vi "Sorting_Single_Frame_Displ_2.vi"(0 "[IN] (X,Y,dX,dY)":dbl[][](array[numeric]), 2 "error IN":errorcluster) -> (3 "[OUT] Displ >1 Frame":dbl[][](array[numeric]), 4 "[OUT] Displ =1 Frame":dbl[][](array[numeric]), 6 "error OUT":errorcluster)   [LabVIEW 2017]
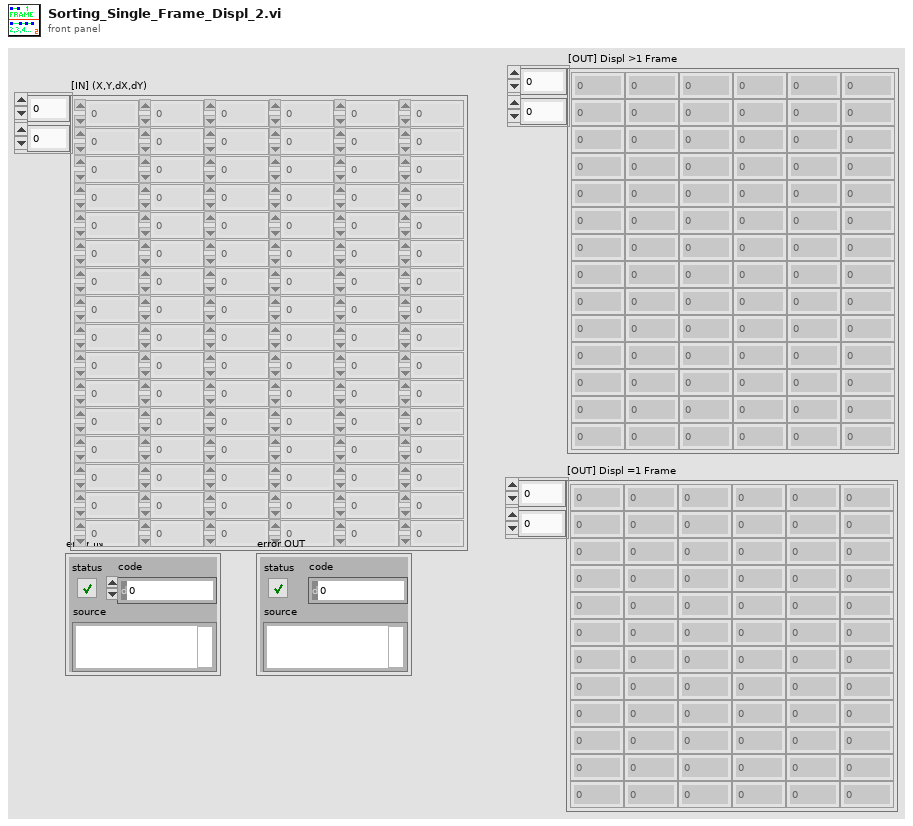
[diagram p1: front panel]
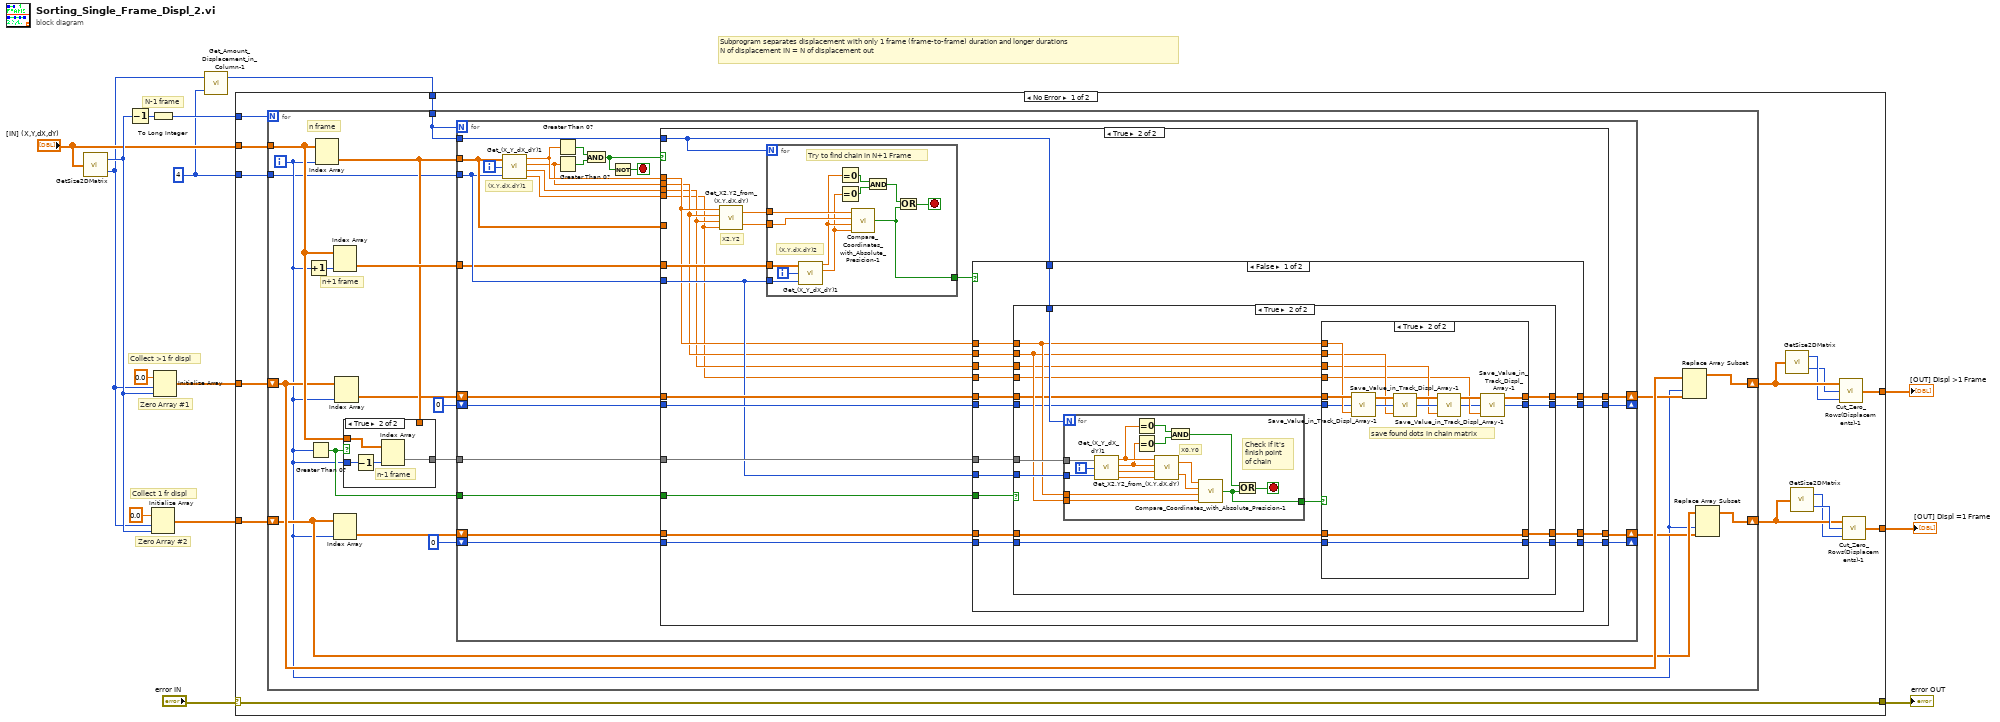
[diagram p0: block diagram]
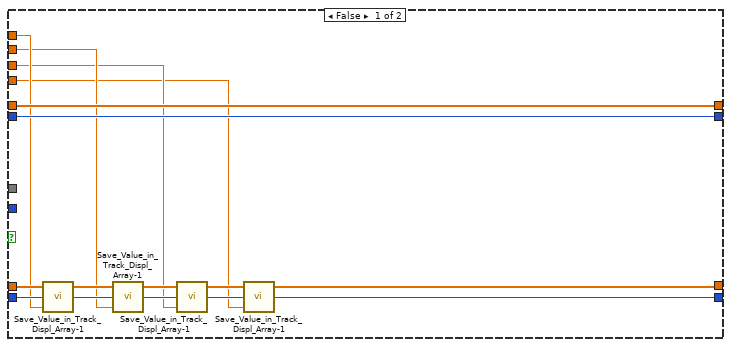
[diagram p4: hidden frame]
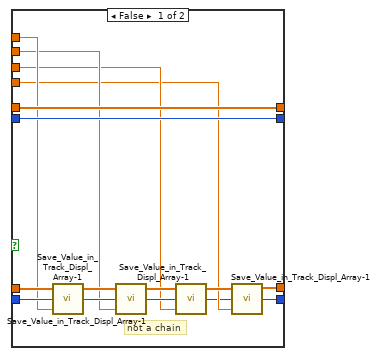
[diagram p5: hidden frame]
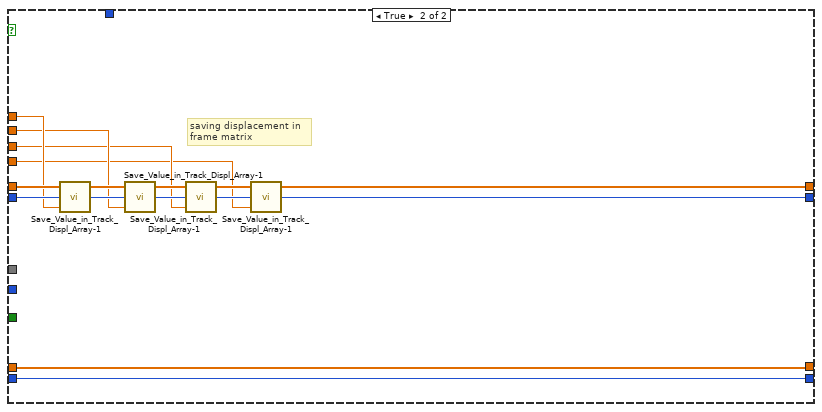
[diagram p6: hidden frame]
diagram:
  w4 = 4 ("y")
  # "Collect >1 fr displ"
  # "Collect 1 fr displ"
  # "Subprogram separates displacement with only 1 frame (frame-to-frame) duration and longer durations\nN of displacement IN = N of displacement out"
  # "Zero Array #2"
  # "Zero Array #1"
  # "N-1 frame"
  n1 = call "GetSize2DMatrix.vi"("Array IN (2D)"="[IN] (X,Y,dX,dY)") -> ("# Cols"=w10:i32, "# Rows"=w5:i32)
  n2 = Decrement(x=w10) -> (x-1=w15:i32)
  n3 = To Long Integer(number=w15) -> (32bit integer=w13:i32)
  n4 = Initialize Array(0.0 ("element"), w5, w10) -> (w9:dbl[][])
  n5 = Initialize Array(0.0 ("element"), w5, w10) -> (w12:dbl[][])
  n6 = call "Get_Amount_Displacement_in_Column-1.vi"("multiplier"=w4, "# Rows"=w5) -> ("Displ amount"=w3:i32)  [unwired: 1 out]
  n7 = case shown="No Error" "error IN" {
    selector: "error IN" -> [w16 w228]
    tunnel: w13 -> [w30 _]
    tunnel: w12 -> [w29 w226]
    tunnel: w9 -> [w28 w227]
    tunnel: "[IN] (X,Y,dX,dY)" -> [w21 _]
    tunnel: [w20 w226] -> w7
    tunnel: [w19 w227] -> w6
    tunnel: w4 -> [w18 _]
    tunnel: w3 -> [w17 _]
    tunnel: [w16 w228] -> w1
    frame No Error {
      n8 = for {
        N: w30 -> [_]
        shift-right: [w38] -> w27
        shift-left: w29 -> [w40]
        shift-right: [w34] -> w23
        shift-left: w28 -> [w36]
        tunnel: w21 -> [w47]
        tunnel: w18 -> [w32]
        tunnel: w17 -> [w31]
        i -> [w33]
        # "n+1 frame"
        # "n frame"
        n9 = Increment(x=w33) -> (x+1=w49:i32)
        n10 = Greater Than 0?(x=w33) -> (x > 0?=w44:bool)
        n11 = Index Array(array=w47, index (col)=w33) -> (element=w45:dbl[])  [unwired: 1 in]
        n12 = Index Array(array=w47, index (col)=w49) -> (element=w48:dbl[])  [unwired: 1 in]
        n13 = Index Array(array=w36, index (col)=w33) -> (element=w42:dbl[])  [unwired: 1 in]
        n14 = Index Array(array=w40, index (col)=w33) -> (element=w43:dbl[])  [unwired: 1 in]
        n15 = case shown="True" w44 {
          tunnel: w47 -> [_ w54]
          tunnel: w33 -> [_ w52]
          tunnel: [w50 w53] -> w46
          tunnel: w45 -> [w50 _]
          frame False {
          }
          frame True {
            # "n-1 frame"
            n16 = Decrement(x=w52) -> (x-1=w51:i32)
            n17 = Index Array(array=w54, index (col)=w51) -> (element=w53:dbl[])  [unwired: 1 in]
          }
        }
        n18 = for {
          N: w31 -> [_]
          tunnel: w48 -> [w67]
          tunnel: w32 -> [w72]
          tunnel: w31 -> [w74]
          tunnel: w45 -> [w73]
          tunnel: w46 -> [w59]
          tunnel: w44 -> [w64]
          shift-right: [w61] -> w39
          shift-left: w43 -> [w62]
          shift-right: [w55] -> w35
          shift-left: w42 -> [w58]
          shift-right: [w60] -> _
          shift-left: 0 -> [w63]
          shift-right: [w56] -> _
          shift-left: 0 -> [w57]
          i -> [w77]
          stop <- w66 stop-if-true
          # "(X,Y,dX,dY)1"
          n19 = call "Get_(X_Y_dX_dY)1.vi"("(X,Y,dX,dY)"=w73, "index"=w77, "multiplier"=w72) -> ("X"=w71:dbl, "Y"=w70:dbl, "dX"=w69:dbl, "dY"=w68:dbl)
          n20 = Greater Than 0?(x=w71) -> (x > 0?=w76:bool)
          n21 = Greater Than 0?(x=w70) -> (x > 0?=w75:bool)
          n22 = And(x=w76, y=w75) -> (x .and. y?=w65:bool)
          n23 = Not(x=w65) -> (.not. x?=w66:bool)
          n24 = case shown="True" w65 {
            tunnel: w74 -> [_ w88]
            tunnel: w73 -> [_ _]
            tunnel: w72 -> [_ w89]
            tunnel: w71 -> [_ w87]
            tunnel: w70 -> [_ w84]
            tunnel: w69 -> [_ w83]
            tunnel: w68 -> [_ w82]
            tunnel: w67 -> [_ w101]
            tunnel: w64 -> [_ w97]
            tunnel: w63 -> [w80 w98]
            tunnel: w62 -> [w81 w99]
            tunnel: [w81 w92] -> w61
            tunnel: [w80 w91] -> w60
            tunnel: w59 -> [_ w90]
            tunnel: w58 -> [w79 w96]
            tunnel: w57 -> [w78 w95]
            tunnel: [w78 w93] -> w56
            tunnel: [w79 w94] -> w55
            frame False {
            }
            frame True {
              # "X2,Y2"
              n25 = call "Get_X2,Y2_from_(X,Y,dX,dY).vi"("dY"=w82, "dX"=w83, "Y1"=w84, "X1"=w87) -> ("Y2 = (Y1+dY)"=w85:dbl, "X2 = (X1+dX)"=w86:dbl)
              n26 = for {
                N: w88 -> [_]
                tunnel: w86 -> [w218]
                tunnel: w85 -> [w217]
                tunnel: w101 -> [w225]
                tunnel: w89 -> [w222]
                tunnel: [w214] -> w100
                i -> [w221]
                stop <- w220 stop-if-true
                # "Try to find chain in N+1 Frame"
                # "(X,Y,dX,dY)2"
                n27 = call "Get_(X_Y_dX_dY)1.vi"("(X,Y,dX,dY)"=w225, "index"=w221, "multiplier"=w222) -> ("X"=w216:dbl, "Y"=w215:dbl)  [unwired: 2 out]
                n28 = Equal To 0?(x=w216) -> (x = 0?=w224:bool)
                n29 = Equal To 0?(x=w215) -> (x = 0?=w223:bool)
                n30 = call "Compare_Coordinates_with_Absolute_Presicion-1.vi"("X 1"=w218, "Y 1"=w217, "X 2"=w216, "Y 2"=w215) -> ("[OUT] Same coordinates?"=w214:bool)  [unwired: 1 in]
                n31 = And(x=w224, y=w223) -> (x .and. y?=w219:bool)
                n32 = Or(x=w219, y=w214) -> (x .or. y?=w220:bool)
              }
              n33 = case shown="False" w100 {
                tunnel: w87 -> [w111 w209]
                tunnel: w83 -> [w109 w203]
                tunnel: w84 -> [w110 w206]
                tunnel: w82 -> [w108 w200]
                tunnel: w99 -> [w116 w211]
                tunnel: w98 -> [w115 w210]
                tunnel: w97 -> [w117 _]
                tunnel: w96 -> [w114 w213]
                tunnel: w95 -> [w113 w212]
                tunnel: [w112 w213] -> w94
                tunnel: [w107 w212] -> w93
                tunnel: [w106 w199] -> w92
                tunnel: [w105 w198] -> w91
                tunnel: w90 -> [w104 _]
                tunnel: w89 -> [w103 _]
                tunnel: w88 -> [w102 _]
                frame False {
                  n34 = case shown="True" w117 {
                    tunnel: w116 -> [w133 w141]
                    tunnel: w115 -> [w132 w140]
                    tunnel: [w133 w139] -> w106
                    tunnel: [w132 w138] -> w105
                    tunnel: w114 -> [w131 w137]
                    tunnel: w113 -> [w130 w136]
                    tunnel: [w119 w135] -> w112
                    tunnel: w111 -> [w129 w145]
                    tunnel: w110 -> [w126 w144]
                    tunnel: w109 -> [w123 w143]
                    tunnel: w108 -> [w120 w142]
                    tunnel: [w118 w134] -> w107
                    tunnel: w104 -> [_ w149]
                    tunnel: w103 -> [_ w148]
                    tunnel: w102 -> [_ w147]
                    frame False {
                      n35 = call "Save_Value_in_Track_Displ_Array-1.vi"("[IN] Value"=w129, "[IN] Index"=w130, "[IN] Empty tracks\nfor points saving"=w131) -> ("[OUT] Index ++"=w127:i32, "[OUT Track with saved value"=w128:dbl[])  [unwired: 1 in]
                      n36 = call "Save_Value_in_Track_Displ_Array-1.vi"("[IN] Value"=w126, "[IN] Index"=w127, "[IN] Empty tracks\nfor points saving"=w128) -> ("[OUT] Index ++"=w124:i32, "[OUT Track with saved value"=w125:dbl[])  [unwired: 1 in]
                      n37 = call "Save_Value_in_Track_Displ_Array-1.vi"("[IN] Value"=w123, "[IN] Index"=w124, "[IN] Empty tracks\nfor points saving"=w125) -> ("[OUT] Index ++"=w121:i32, "[OUT Track with saved value"=w122:dbl[])  [unwired: 1 in]
                      n38 = call "Save_Value_in_Track_Displ_Array-1.vi"("[IN] Value"=w120, "[IN] Index"=w121, "[IN] Empty tracks\nfor points saving"=w122) -> ("[OUT] Index ++"=w118:i32, "[OUT Track with saved value"=w119:dbl[])  [unwired: 1 in]
                    }
                    frame True {
                      n39 = for {
                        N: w147 -> [_]
                        tunnel: w149 -> [w197]
                        tunnel: w148 -> [w195]
                        tunnel: w145 -> [w184]
                        tunnel: w144 -> [w183]
                        tunnel: [w182] -> w146
                        i -> [w196]
                        stop <- w191 stop-if-true
                        # "Check if it's \nfinish point\nof chain"
                        # "X0,Y0"
                        n40 = call "Get_(X_Y_dX_dY)1.vi"("(X,Y,dX,dY)"=w197, "index"=w196, "multiplier"=w195) -> ("X"=w190:dbl, "Y"=w189:dbl, "dX"=w188:dbl, "dY"=w187:dbl)
                        n41 = Equal To 0?(x=w190) -> (x = 0?=w194:bool)
                        n42 = Equal To 0?(x=w189) -> (x = 0?=w193:bool)
                        n43 = call "Get_X2,Y2_from_(X,Y,dX,dY).vi"("dY"=w187, "dX"=w188, "Y1"=w189, "X1"=w190) -> ("Y2 = (Y1+dY)"=w185:dbl, "X2 = (X1+dX)"=w186:dbl)
                        n44 = And(x=w194, y=w193) -> (x .and. y?=w192:bool)
                        n45 = call "Compare_Coordinates_with_Absolute_Presicion-1.vi"("X 1"=w186, "Y 1"=w185, "X 2"=w184, "Y 2"=w183) -> ("[OUT] Same coordinates?"=w182:bool)  [unwired: 1 in]
                        n46 = Or(x=w192, y=w182) -> (x .or. y?=w191:bool)
                      }
                      n47 = case shown="True" w146 {
                        tunnel: w145 -> [w161 w178]
                        tunnel: w144 -> [w158 w174]
                        tunnel: w143 -> [w155 w171]
                        tunnel: w142 -> [w153 w169]
                        tunnel: w141 -> [w165 w179]
                        tunnel: w140 -> [w164 w177]
                        tunnel: [w165 w167] -> w139
                        tunnel: [w164 w166] -> w138
                        tunnel: w137 -> [w163 w181]
                        tunnel: w136 -> [w162 w180]
                        tunnel: [w151 w181] -> w135
                        tunnel: [w150 w180] -> w134
                        frame False {
                          # "not a chain"
                          n48 = call "Save_Value_in_Track_Displ_Array-1.vi"("[IN] Value"=w161, "[IN] Index"=w162, "[IN] Empty tracks\nfor points saving"=w163) -> ("[OUT] Index ++"=w159:i32, "[OUT Track with saved value"=w160:dbl[])  [unwired: 1 in]
                          n49 = call "Save_Value_in_Track_Displ_Array-1.vi"("[IN] Value"=w158, "[IN] Index"=w159, "[IN] Empty tracks\nfor points saving"=w160) -> ("[OUT] Index ++"=w156:i32, "[OUT Track with saved value"=w157:dbl[])  [unwired: 1 in]
                          n50 = call "Save_Value_in_Track_Displ_Array-1.vi"("[IN] Value"=w155, "[IN] Index"=w156, "[IN] Empty tracks\nfor points saving"=w157) -> ("[OUT] Index ++"=w152:i32, "[OUT Track with saved value"=w154:dbl[])  [unwired: 1 in]
                          n51 = call "Save_Value_in_Track_Displ_Array-1.vi"("[IN] Value"=w153, "[IN] Index"=w152, "[IN] Empty tracks\nfor points saving"=w154) -> ("[OUT] Index ++"=w150:i32, "[OUT Track with saved value"=w151:dbl[])  [unwired: 1 in]
                        }
                        frame True {
                          # "save found dots in chain matrix"
                          n52 = call "Save_Value_in_Track_Displ_Array-1.vi"("[IN] Value"=w178, "[IN] Index"=w177, "[IN] Empty tracks\nfor points saving"=w179) -> ("[OUT] Index ++"=w175:i32, "[OUT Track with saved value"=w176:dbl[])  [unwired: 1 in]
                          n53 = call "Save_Value_in_Track_Displ_Array-1.vi"("[IN] Value"=w174, "[IN] Index"=w175, "[IN] Empty tracks\nfor points saving"=w176) -> ("[OUT] Index ++"=w172:i32, "[OUT Track with saved value"=w173:dbl[])  [unwired: 1 in]
                          n54 = call "Save_Value_in_Track_Displ_Array-1.vi"("[IN] Value"=w171, "[IN] Index"=w172, "[IN] Empty tracks\nfor points saving"=w173) -> ("[OUT] Index ++"=w168:i32, "[OUT Track with saved value"=w170:dbl[])  [unwired: 1 in]
                          n55 = call "Save_Value_in_Track_Displ_Array-1.vi"("[IN] Value"=w169, "[IN] Index"=w168, "[IN] Empty tracks\nfor points saving"=w170) -> ("[OUT] Index ++"=w166:i32, "[OUT Track with saved value"=w167:dbl[])  [unwired: 1 in]
                        }
                      }
                    }
                  }
                }
                frame True {
                  # "saving displacement in \nframe matrix"
                  n56 = call "Save_Value_in_Track_Displ_Array-1.vi"("[IN] Value"=w209, "[IN] Index"=w210, "[IN] Empty tracks\nfor points saving"=w211) -> ("[OUT] Index ++"=w207:i32, "[OUT Track with saved value"=w208:dbl[])  [unwired: 1 in]
                  n57 = call "Save_Value_in_Track_Displ_Array-1.vi"("[IN] Value"=w206, "[IN] Index"=w207, "[IN] Empty tracks\nfor points saving"=w208) -> ("[OUT] Index ++"=w204:i32, "[OUT Track with saved value"=w205:dbl[])  [unwired: 1 in]
                  n58 = call "Save_Value_in_Track_Displ_Array-1.vi"("[IN] Value"=w203, "[IN] Index"=w204, "[IN] Empty tracks\nfor points saving"=w205) -> ("[OUT] Index ++"=w201:i32, "[OUT Track with saved value"=w202:dbl[])  [unwired: 1 in]
                  n59 = call "Save_Value_in_Track_Displ_Array-1.vi"("[IN] Value"=w200, "[IN] Index"=w201, "[IN] Empty tracks\nfor points saving"=w202) -> ("[OUT] Index ++"=w198:i32, "[OUT Track with saved value"=w199:dbl[])  [unwired: 1 in]
                }
              }
            }
          }
        }
        n60 = Replace Array Subset(array=w40, new element=w39, index (col)=w33) -> (w38:dbl[][])  [unwired: 1 in]
        n61 = Replace Array Subset(array=w36, new element=w35, index (col)=w33) -> (w34:dbl[][])  [unwired: 1 in]
      }
      n62 = call "GetSize2DMatrix.vi"("Array IN (2D)"=w27) -> ("# Cols"=w26:i32, "# Rows"=w25:i32)
      n63 = call "GetSize2DMatrix.vi"("Array IN (2D)"=w23) -> ("# Cols"=w22:i32, "# Rows"=w24:i32)
      n64 = call "Cut_Zero_Rows(Displacements)-1.vi"("# Cols"=w26, "# Rows"=w25, "Array IN"=w27) -> ("Array OUT"=w20:dbl[][])
      n65 = call "Cut_Zero_Rows(Displacements)-1.vi"("# Cols"=w22, "# Rows"=w24, "Array IN"=w23) -> ("Array OUT"=w19:dbl[][])
    }
    frame Error {
    }
  }
  "[OUT] Displ >1 Frame" <- w7
  "[OUT] Displ =1 Frame" <- w6
  "error OUT" <- w1
